vi "LVH5Sget_select_pointlist.vi"(6 "error in (no error)":errorcluster, 7 "Numpoints (All)":i64=-1, 8 "Start (0)":u64, 9 "HDF5 Space Ref":T1) -> (0 "error out":errorcluster, 2 "Pointlist":u64[][](array[numeric]), 3 "HDF5 Ref out":T1)   [LabVIEW 2017]
doc: "Returns a list of the points selected in a dataspace"
uses:
  <vilib>/UPVI/lvhdf5/library.llb/HDF5 Ref.ctl
  <vilib>/UPVI/lvhdf5/h5helper.dll
panel:
  # "LVHDF5 Toolkit\nCopyright (c) 2005-2013 by Jason D. Sommerville\nCopyright (c) 2014 by UPVI, LLC.\n\nThis use and distribution of this file is governed by the terms found in \nLICENSE.txt distributed with this toolkit and installed at\n <user.lib>\\_lvhdf5\\LICENSE.txt"
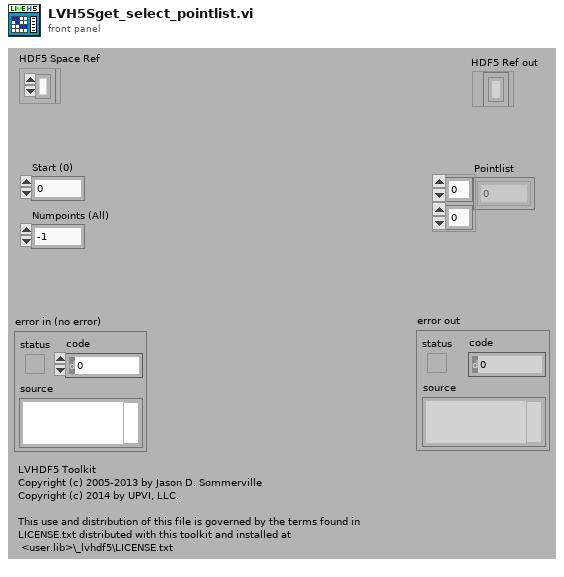
[diagram p1: front panel]
types:
  T1 = typedef "HDF5 Ref.ctl" = refnum<k1>
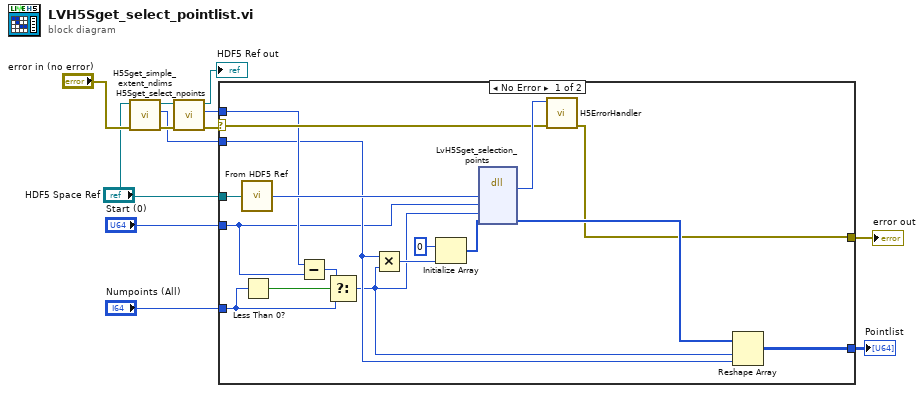
[diagram p0: block diagram]
diagram:
  n1 = call <vilib>:"H5Sget_simple_extent_ndims.vi"("error in (no error)"="error in (no error)", "HDF5 Space Ref"="HDF5 Space Ref") -> ("error out"=w5:errorcluster, "Rank"=w2:i32, "HDF5 Ref out"=w3:T1)  [unwired: 5 in]
  n2 = call <vilib>:"H5Sget_select_npoints.vi"("error in (no error)"=w5, "HDF5 Space Ref"=w3) -> ("error out"=w9:errorcluster, "Count"=w7:i64, "HDF5 Ref out"=→"HDF5 Ref out":T1)  [unwired: 5 in]
  n3 = case shown="No Error" w9 {
    selector: w9 -> [w26 w30]
    tunnel: [w14 w30] -> w12
    tunnel: "HDF5 Space Ref" -> [w29 _]
    tunnel: "Start (0)" -> [w16 _]
    tunnel: "Numpoints (All)" -> [w23 _]
    tunnel: w7 -> [w24 _]
    tunnel: w2 -> [w17 _]
    tunnel: [w18 _] -> w1
    frame No Error {
      n4 = call <vilib>:"From HDF5 Ref.vi"("HDF5 Ref"=w29) -> ("I32"=w28:i32)
      n5 = Less Than 0?(x=w23) -> (x < 0?=w25:bool)
      n6 = Subtract(x=w24, y=w16) -> (x-y=w22:u64)
      n7 = Select(t=w22, s=w25, f=w23) -> (s? t:f=w13:u64)
      n8 = Multiply(x=w17, y=w13) -> (x*y=w19:u64)
      n9 = Initialize Array(u64 0 ("element"), w19) -> (w20:u64[])
      n10 = dll-call lib="C:/Program Files/National Instruments/LabVIEW 2017/vi.lib/UPVI/lvhdf5/h5helper.dll" fn="LvH5Sget_selection_points"("space_id"=w28, "startpoint"=w16, "numpoints"=w13, "pointlist"=w20) -> ("return type"=w27:i32, "pointlist"=w15:u64[])  [unwired: 6 in, 2 out]
      n11 = call <vilib>:"H5ErrorHandler.vi"("error in (no error)"=w26, "herr_t"=w27) -> ("error out"=w14:errorcluster)  [unwired: 3 in, 4 out]
      n12 = Reshape Array(w15, w13, w17) -> (w18:u64[][])
    }
    frame Error {
    }
  }
  "error out" <- w12
  "Pointlist" <- w1
